vi "PubSub.vi"() -> ()   [LabVIEW 2025]
uses:
  libzmq-v143-mt-4_3_6/ctls/SocketType.ctl
  libzmq-v143-mt-4_3_6/ctls/SocketOption.ctl
  zeromq/Receive_string.vi
  zeromq/Send_string.vi
  zeromq/Context.lvclass
  libzmq-v143-mt-4_3_6/LibZMQ.lvlib
  zeromq/Socket.lvclass
panel:
  out "data 2":string
  out "data":string
  out "error out 2":errorcluster
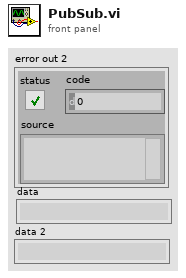
[diagram p1: front panel]
types:
  T1 = typedef "LibZMQ.lvlib/SocketOption.ctl" = enum8{"NONE", "ZMQ_HWM", "<2>", "ZMQ_SWAP", "ZMQ_AFFINITY", "ZMQ_ROUTING_ID", "ZMQ_SUBSCRIBE", "ZMQ_UNSUBSCRIBE", "ZMQ_RATE", "ZMQ_RECOVERY_IVL", "ZMQ_MCAST_LOOP", "ZMQ_SNDBUF", "ZMQ_RCVBUF", "ZMQ_RCVMORE", "ZMQ_FD", "ZMQ_EVENTS", "ZMQ_TYPE", "ZMQ_LINGER", "ZMQ_RECONNECT_IVL", "ZMQ_BACKLOG", "ZMQ_RECOVERY_IVL_MSEC", "ZMQ_RECONNECT_IVL_MAX", "ZMQ_MAXMSGSIZE", "ZMQ_SNDHWM", "ZMQ_RCVHWM", "ZMQ_MULTICAST_HOPS", "<26>", "ZMQ_RCVTIMEO", "ZMQ_SNDTIMEO", "<29>", "<30>", "ZMQ_IPV4ONLY", "ZMQ_LAST_ENDPOINT", "ZMQ_ROUTER_MANDATORY", "ZMQ_TCP_KEEPALIVE", "ZMQ_TCP_KEEPALIVE_CNT", "ZMQ_TCP_KEEPALIVE_IDLE", "ZMQ_TCP_KEEPALIVE_INTVL", "ZMQ_TCP_ACCEPT_FILTER", "ZMQ_IMMEDIATE", "ZMQ_XPUB_VERBOSE", "ZMQ_ROUTER_RAW", "ZMQ_IPV6", "ZMQ_MECHANISM", "ZMQ_PLAIN_SERVER", "ZMQ_PLAIN_USERNAME", "ZMQ_PLAIN_PASSWORD", "ZMQ_CURVE_SERVER", "ZMQ_CURVE_PUBLICKEY", "ZMQ_CURVE_SECRETKEY", "ZMQ_CURVE_SERVERKEY", "ZMQ_PROBE_ROUTER", "ZMQ_REQ_CORRELATE", "ZMQ_REQ_RELAXED", "ZMQ_CONFLATE", "ZMQ_ZAP_DOMAIN", "ZMQ_ROUTER_HANDOVER", "ZMQ_TOS", "ZMQ_IPC_FILTER_PID", "ZMQ_IPC_FILTER_UID", "ZMQ_IPC_FILTER_GID", "ZMQ_CONNECT_ROUTING_ID", "ZMQ_GSSAPI_SERVER", "ZMQ_GSSAPI_PRINCIPAL", "ZMQ_GSSAPI_SERVICE_PRINCIPAL", "ZMQ_GSSAPI_PLAINTEXT", "ZMQ_HANDSHAKE_IVL", "<67>", "ZMQ_SOCKS_PROXY", "ZMQ_XPUB_NODROP", "ZMQ_BLOCKY", "ZMQ_XPUB_MANUAL", "ZMQ_XPUB_WELCOME_MSG", "ZMQ_STREAM_NOTIFY", "ZMQ_INVERT_MATCHING", "ZMQ_HEARTBEAT_IVL", "ZMQ_HEARTBEAT_TTL", "ZMQ_HEARTBEAT_TIMEOUT", "ZMQ_XPUB_VERBOSER", "ZMQ_CONNECT_TIMEOUT", "ZMQ_TCP_MAXRT", "ZMQ_THREAD_SAFE", "<82>", "<83>", "ZMQ_MULTICAST_MAXTPDU", "ZMQ_VMCI_BUFFER_SIZE", "ZMQ_VMCI_BUFFER_MIN_SIZE", "ZMQ_VMCI_BUFFER_MAX_SIZE", "ZMQ_VMCI_CONNECT_TIMEOUT", "ZMQ_USE_FD", "ZMQ_GSSAPI_PRINCIPAL_NAMETYPE", "ZMQ_GSSAPI_SERVICE_PRINCIPAL_NAMETYPE", "ZMQ_BINDTODEVICE", "ZMQ_ZAP_ENFORCE_DOMAIN", "ZMQ_LOOPBACK_FASTPATH", "ZMQ_METADATA", "ZMQ_MULTICAST_LOOP", "ZMQ_ROUTER_NOTIFY"}
  T2 = typedef "LibZMQ.lvlib/SocketType.ctl" = enum8{"PAIR", "PUB", "SUB", "REQ", "REP", "DEALER", "ROUTER", "PULL", "PUSH", "XPUB", "XSUB", "STREAM"}
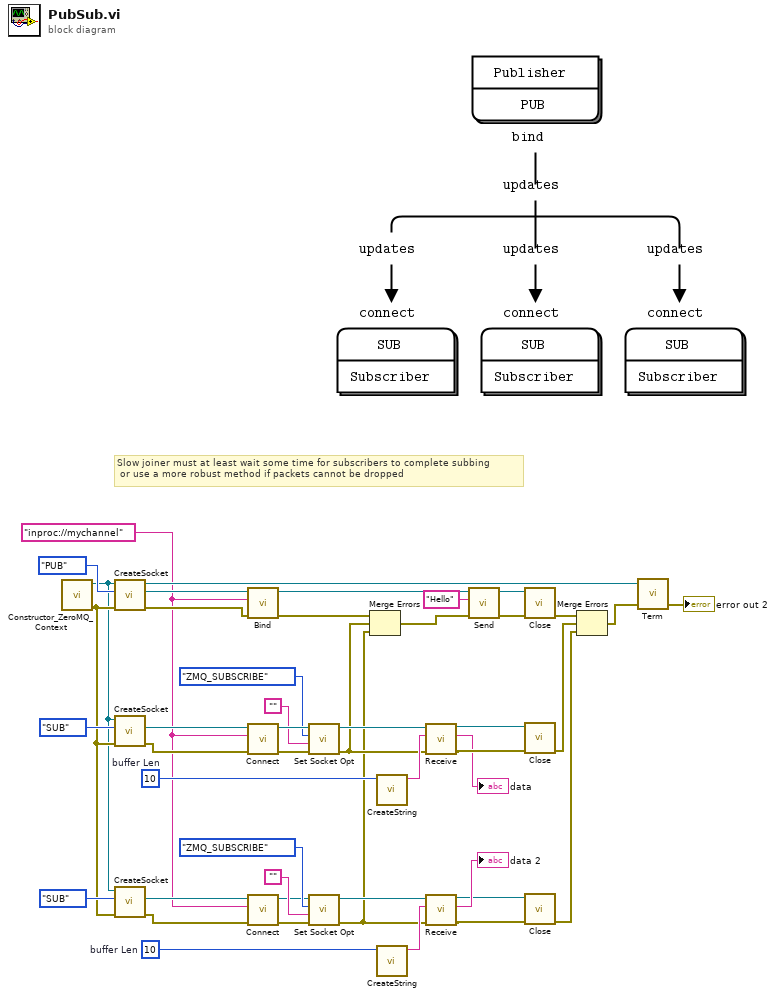
[diagram p0: block diagram]
diagram:
  w13 = 10  # buffer Len
  w32 = 10  # buffer Len
  w1 = "inproc://mychannel"
  # "Slow joiner must at least wait some time for subscribers to complete subbing\n or use a more robust method if packets cannot be dropped"
  n1 = call "Constructor_ZeroMQ_Context.vi"() -> ("error out"=w8:errorcluster, "context out"=w7:refnum<class "Context.lvclass">)  [unwired: 10 in]
  n2 = call "CreateSocket.vi"("error in"=w8, "Socket Type"=SocketType."PUB", "context in"=w7) -> ("error out"=w27:errorcluster, "socket out"=w46:refnum<class "Socket.lvclass">, "context out"=w38:refnum<class "Context.lvclass">)  [unwired: 6 in]
  n3 = call "CreateSocket.vi"("error in"=w8, "Socket Type"=SocketType."SUB", "context in"=w7) -> ("error out"=w43:errorcluster, "socket out"=w44:refnum<class "Socket.lvclass">)  [unwired: 6 in, 1 out]
  n4 = call "CreateSocket.vi"("error in"=w8, "Socket Type"=SocketType."SUB", "context in"=w7) -> ("error out"=w10:errorcluster, "socket out"=w9:refnum<class "Socket.lvclass">)  [unwired: 6 in, 1 out]
  n5 = call "Bind.vi"("error in"=w27, "endpoint"=w1, "socket in"=w46) -> ("error out"=w6:errorcluster, "socket out"=w34:refnum<class "Socket.lvclass">)  [unwired: 7 in]
  n6 = call "Connect.vi"("error in"=w43, "endpoint"=w1, "socket in"=w44) -> ("error out"=w24:errorcluster, "socket out"=w26:refnum<class "Socket.lvclass">)  [unwired: 7 in]
  n7 = call "Connect.vi"("error in"=w10, "endpoint"=w1, "socket in"=w9) -> ("error out"=w19:errorcluster, "socket out"=w17:refnum<class "Socket.lvclass">)  [unwired: 7 in]
  n8 = call "Set Socket Opt.vi"("error in"=w24, "value"="", "Socket option"=SocketOption."ZMQ_SUBSCRIBE", "socket in"=w26) -> ("error out"=w4:errorcluster, "socket out"=w25:refnum<class "Socket.lvclass">)  [unwired: 6 in]
  n9 = call "Set Socket Opt.vi"("error in"=w19, "value"="", "Socket option"=SocketOption."ZMQ_SUBSCRIBE", "socket in"=w17) -> ("error out"=w3:errorcluster, "socket out"=w18:refnum<class "Socket.lvclass">)  [unwired: 6 in]
  n10 = Merge Errors(w6, w4, w3) -> (w5:errorcluster)
  n11 = call "CreateString.vi"("length"=w32) -> ("string"=w33:string)  [unwired: 10 in]
  n12 = call "CreateString.vi"("length"=w13) -> ("string"=w12:string)  [unwired: 10 in]
  n13 = call-poly "Receive.vi"("error in"=w4, "buf in"=w33, "socket in"=w25) -> ("error out"=w30:errorcluster, "data"=→"data":string, "socket out"=w31:refnum<class "Socket.lvclass">)  [unwired: 6 in]
  n14 = call-poly "Receive.vi"("error in"=w3, "buf in"=w12, "socket in"=w18) -> ("error out"=w15:errorcluster, "data"=→"data 2":string, "socket out"=w14:refnum<class "Socket.lvclass">)  [unwired: 6 in]
  n15 = call-poly "Send.vi"("error in"=w5, "data"="Hello", "socket in"=w34) -> ("error out"=w36:errorcluster, "socket out"=w35:refnum<class "Socket.lvclass">)  [unwired: 7 in]
  n16 = call "Close.vi"("error in"=w36, "socket"=w35) -> ("error out"=w41:errorcluster)  [unwired: 9 in]
  n17 = call "Close.vi"("error in"=w30, "socket"=w31) -> ("error out"=w28:errorcluster)  [unwired: 9 in]
  n18 = call "Close.vi"("error in"=w15, "socket"=w14) -> ("error out"=w2:errorcluster)  [unwired: 9 in]
  n19 = Merge Errors(w41, w28, w2) -> (w40:errorcluster)
  n20 = call "Term.vi"("error in"=w40, "context in"=w38) -> ("error out"=→"error out 2":errorcluster)  [unwired: 3 in]
